vi "SvgDoc Set Fill Color.vi"(8 "error in (no error)":errorcluster, 10 "Color":refnum<k24>, 11 "SVG DOC":refnum<k24>) -> (0 "error out":errorcluster, 3 ".NET Refnum out":refnum<k24>)   [LabVIEW 2020, in "SvgDotNet.lvlib"]
uses:
  SvgDotNet.lvlib
  C:/Users/huipeng8/Desktop/SVG.NET/Svg.dll
  Svg.dll
panel:
  # "Connector Pane"
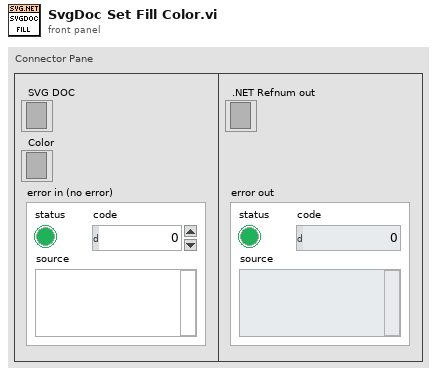
[diagram p1: front panel]
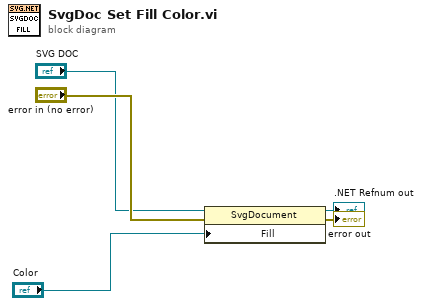
[diagram p0: block diagram]
diagram:
  n1 = property class="SvgDocument"(reference="SVG DOC", error in="error in (no error)", "Fill"="Color") -> (reference out=→".NET Refnum out":refnum<k24>, error out=→"error out":errorcluster)
